vi "Main Loop.vi"() -> ()   [LabVIEW 2011]
panel:
  out "Drone Status Bits.Battery Voltage Too Low?":bool
  out "video data out":string
  in  "index":i32
  out "Navdata Demo":u32
  out "Numeric":u32
  in  "vertical speed":sgl(slide) scale=-1.0..1.0
  in  "yaw":sgl(slide) scale=-1.0..1.0
  in  "pitch":sgl(slide) scale=-1.0..1.0
  in  "roll":sgl(slide) scale=-1.0..1.0
  in  "Land":bool
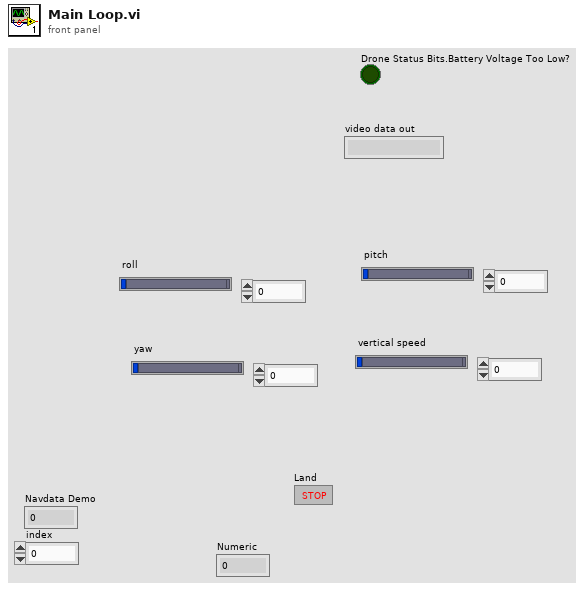
[diagram p1: front panel]
types:
  T1 = enum16{"big-endian, network order", "native, host order", "little-endian"}
  T2 = cluster{"Drone Status Bits":cluster{"Flying?":bool, "Video Enabled?":bool, "Vision Enabled?":bool, "Angular Speed Control?":bool, "Altitude Control?":bool, "Start button?":bool, "Control Command Recieved?":bool, "Trim Command Recieved?":bool, "Trim Running?":bool, "Trim Succeeded?":bool, "Navdata Demo Mode?":bool, "Navdata Bootstrap Mode?":bool, "Motors Com Down?":bool, "Unknown":bool, "Gyrometer Problem?":bool, "Battery Voltage Too Low?":bool, "Battery Voltage Too High?":bool, "Timer Elapsed?":bool, "Power Too Low?":bool, "Angles Out Of Range?":bool, "Too Much Wind?":bool, "Ultrasound Deaf?":bool, "Cutout Detected?":bool, "PIC Version Number OK?":bool, "ATCodec Thread On?":bool, "Navdata Thread On?":bool, "Video Thread On?":bool, "Acquisition Thread On?":bool, "Control Watchdog Delay?":bool, "ADC Watchdog Delay?":bool, "Communications Problem?":bool, "Emergency?":bool}, "Header":u32, "Sequence Number":u32, "Vision Defined?":bool, "Blocks":cluster{"Size":u16, "Data":u8[], "ID":enum16{"NAVDATA_DEMO", "NAVDATA_TIME", "NAVDATA_RAW_MEASURES", "NAVDATA_PHYS_MEASURES", "NAVDATA_GYROS_OFFSETS", "NAVDATA_EULER_ANGLES", "NAVDATA_REFERENCES", "NAVDATA_TRIMS", "NAVDATA_RC_REFERENCES", "NAVDATA_PWM", "NAVDATA_ALTITUDE", "NAVDATA_VISION_RAW", "NAVDATA_VISION_OF", "NAVDATA_VISION", "NAVDATA_VISION_PERF", "NAVDATA_TRACKERS_SEND", "NAVDATA_VISION_DETECT", "NAVDATA_WATCHDOG", "NAVDATA_ADC_DATA_FRAME", "NAVDATA_VIDEO_STREAM", "NAVDATA_GAMES"}}[]}
  T3 = cluster{"Size":u16, "Data":u8[], "ID":enum16{"NAVDATA_DEMO", "NAVDATA_TIME", "NAVDATA_RAW_MEASURES", "NAVDATA_PHYS_MEASURES", "NAVDATA_GYROS_OFFSETS", "NAVDATA_EULER_ANGLES", "NAVDATA_REFERENCES", "NAVDATA_TRIMS", "NAVDATA_RC_REFERENCES", "NAVDATA_PWM", "NAVDATA_ALTITUDE", "NAVDATA_VISION_RAW", "NAVDATA_VISION_OF", "NAVDATA_VISION", "NAVDATA_VISION_PERF", "NAVDATA_TRACKERS_SEND", "NAVDATA_VISION_DETECT", "NAVDATA_WATCHDOG", "NAVDATA_ADC_DATA_FRAME", "NAVDATA_VIDEO_STREAM", "NAVDATA_GAMES"}}[]
  T4 = enum16{"NAVDATA_DEMO", "NAVDATA_TIME", "NAVDATA_RAW_MEASURES", "NAVDATA_PHYS_MEASURES", "NAVDATA_GYROS_OFFSETS", "NAVDATA_EULER_ANGLES", "NAVDATA_REFERENCES", "NAVDATA_TRIMS", "NAVDATA_RC_REFERENCES", "NAVDATA_PWM", "NAVDATA_ALTITUDE", "NAVDATA_VISION_RAW", "NAVDATA_VISION_OF", "NAVDATA_VISION", "NAVDATA_VISION_PERF", "NAVDATA_TRACKERS_SEND", "NAVDATA_VISION_DETECT", "NAVDATA_WATCHDOG", "NAVDATA_ADC_DATA_FRAME", "NAVDATA_VIDEO_STREAM", "NAVDATA_GAMES"}
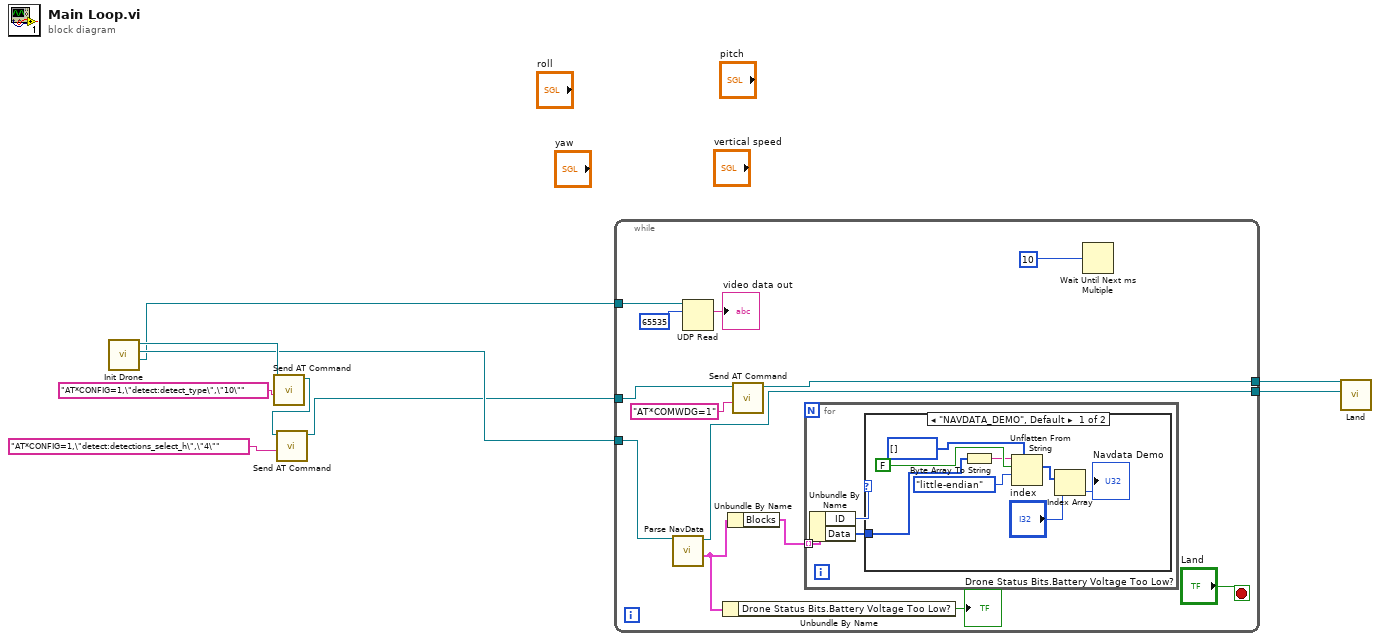
[diagram p0: block diagram]
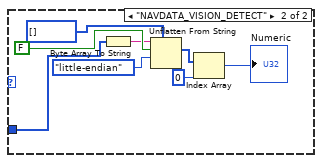
[diagram p2: hidden frame]
diagram:
  n1 = call "Init Drone.vi"() -> ("Video Interface"=w1:refnum<k16>, "NavData Port"=w8:refnum<k16>, "AT Command Port"=w9:refnum<k16>)  [unwired: 9 in]
  n2 = call "Send AT Command.vi"("AT Command"="AT*CONFIG=1,\"detect:detect_type\",\"10\"", "AT Command Port"=w9) -> ("AT Command Port"=w6:refnum<k16>)  [unwired: 9 in]
  n3 = call "Send AT Command.vi"("AT Command"="AT*CONFIG=1,\"detect:detections_select_h\",\"4\"", "AT Command Port"=w6) -> ("AT Command Port"=w4:refnum<k16>)  [unwired: 9 in]
  n4 = while {
    tunnel: w8 -> [w16]
    tunnel: [w18] -> w3
    tunnel: w4 -> [w19]
    tunnel: [w15] -> w2
    tunnel: w1 -> [w14]
    stop <- "Land" stop-if-true
    n5 = call "Parse NavData.vi"("NavData Port"=w16) -> ("NavData"=w11:T2, "NavData Port"=w15:refnum<k16>)  [unwired: 9 in]
    n6 = UDP Read(connection ID=w14, max size (548)=65535) -> (data out=→"video data out":string)  [unwired: 2 in, 4 out]
    n7 = Unbundle By Name(w11) -> ("Drone Status Bits.Battery Voltage Too Low?"=→"Drone Status Bits.Battery Voltage Too Low?":bool)
    n8 = Unbundle By Name(w11) -> ("Blocks"=w20:T3)
    n9 = call "Send AT Command.vi"("AT Command"="AT*COMWDG=1", "AT Command Port"=w19) -> ("AT Command Port"=w18:refnum<k16>)  [unwired: 9 in]
    n10 = for {
      tunnel: w20 -> [w25] mode=indexing
      n11 = Unbundle By Name(w25) -> ("ID"=w24:T4, "Data"=w23:u8[])
      n12 = case shown="\"NAVDATA_DEMO\", Default" w24 {
        tunnel: w23 -> [w27 w38]
        frame "NAVDATA_DEMO", Default {
          n13 = Byte Array To String(unsigned byte array=w27) -> (string=w31:string)
          n14 = Unflatten From String(type=u32[] [], binary string=w31, data includes array or string size? (T)=FALSE, byte order (0:big-endian, network order)=T1."little-endian") -> (value=w28:u32[])  [unwired: 1 in, 2 out]
          n15 = Index Array(array=w28, index="index") -> (element=→"Navdata Demo":u32)
        }
        frame "NAVDATA_VISION_DETECT" {
          n16 = Byte Array To String(unsigned byte array=w38) -> (string=w39:string)
          n17 = Unflatten From String(type=u32[] [], binary string=w39, data includes array or string size? (T)=FALSE, byte order (0:big-endian, network order)=T1."little-endian") -> (value=w35:u32[])  [unwired: 1 in, 2 out]
          n18 = Index Array(array=w35, index=0) -> (element=→"Numeric":u32)
        }
      }
    }
    n19 = Wait Until Next ms Multiple(millisecond multiple=u32 10) -> ()  [unwired: 1 out]
  }
  n20 = call "Land.vi"("NavData Port"=w2, "AT Command Port"=w3) -> ()  [unwired: 8 in, 2 out]
